vi "Write Floating Number Format.vi"(8 "error in (no error)":errorcluster, 10 "Floating Number Format":string, 11 "Serializer.openg-ini in":refnum<class "Serializer.openg-ini.lvclass">) -> (0 "error out":errorcluster, 3 "Serializer.openg-ini out":refnum<class "Serializer.openg-ini.lvclass">)   [LabVIEW 2019, in "OpenSerializer.OpenG-ini.lvlib" / "Serializer.openg-ini.lvclass"]
uses:
  Serializer.openg-ini.lvclass
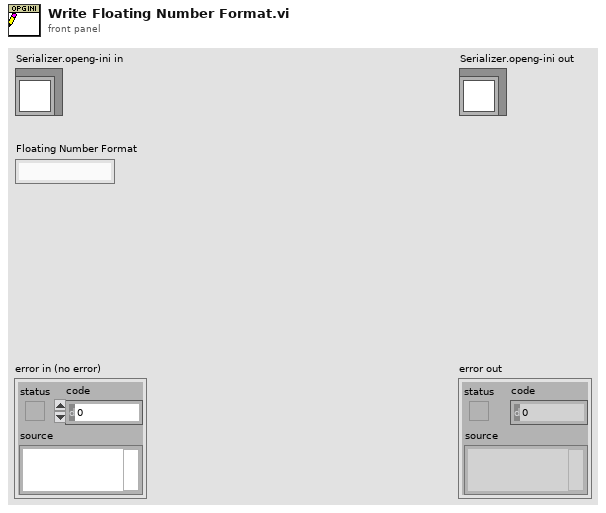
[diagram p1: front panel]
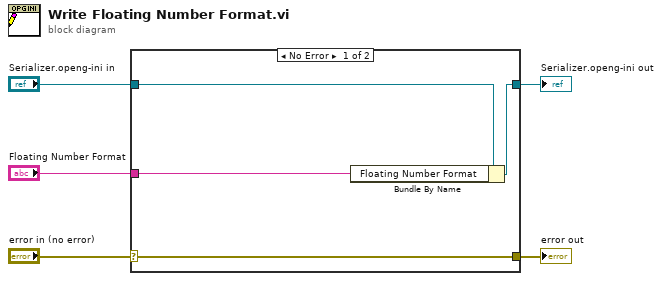
[diagram p0: block diagram]
diagram:
  n1 = case shown="No Error" "error in (no error)" {
    selector: "error in (no error)" -> [w9 w10]
    tunnel: [w9 w10] -> w4
    tunnel: [w7 w11] -> w2
    tunnel: "Serializer.openg-ini in" -> [w8 w11]
    tunnel: "Floating Number Format" -> [w6 _]
    frame No Error {
      n2 = Bundle By Name(cluster=w8, "Floating Number Format"=w6) -> (w7:refnum<class "Serializer.openg-ini.lvclass">)
    }
    frame Error {
    }
  }
  "error out" <- w4
  "Serializer.openg-ini out" <- w2
